vi "setTextToDocument.vi"(8 "error in (no error)":errorcluster, 11 "xwpfRun in":refnum<class "xwpfRun.lvclass">) -> (0 "error out":errorcluster, 3 "xwpfRun out":refnum<class "xwpfRun.lvclass">)   [LabVIEW 2017, in "Word_Specific.lvlib" / "xwpfRun.lvclass"]
uses:
  xwpfRun.lvclass
  xwpfRun.lvclass/xwpfRun.ctl
  C:/Program Files (x86)/National Instruments/LabVIEW 2017/vi.lib/BenjaminR/LabVIEW NPOI/lib/NPOI 2.1.1/NPOI.OOXML.dll
  Program Files (x86)/National Instruments/LabVIEW 2017/vi.lib/BenjaminR/LabVIEW NPOI/lib/NPOI 2.1.1/NPOI.OOXML.dll
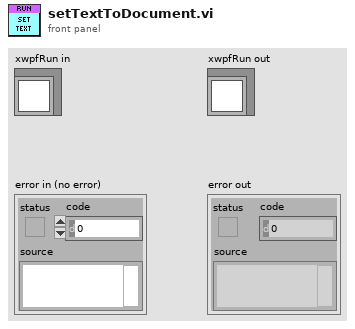
[diagram p1: front panel]
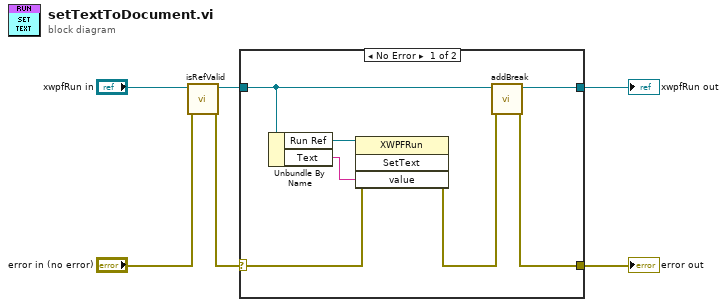
[diagram p0: block diagram]
diagram:
  n1 = call-dynamic "isRefValid.vi"("error in (no error)"="error in (no error)", "xwpfRun in"="xwpfRun in") -> ("error out"=w1:errorcluster, "xwpfRun out"=w3:refnum<class "xwpfRun.lvclass">)  [unwired: 8 in]
  n2 = case shown="No Error" w1 {
    selector: w1 -> [w11 w15]
    tunnel: [w7 w15] -> w6
    tunnel: [w9 w14] -> w4
    tunnel: w3 -> [w12 w14]
    frame No Error {
      n3 = Unbundle By Name(w12) -> ("Run Ref"=w13:refnum<k24>, "Text"=w10:string)
      n4 = invoke class="XWPFRun" method="SetText"(reference=w13, error in=w11, "value"=w10) -> (error out=w8:errorcluster)  [unwired: 1 in, 3 out]
      n5 = call-dynamic "addBreak.vi"("error in (no error)"=w8, "xwpfRun in"=w12) -> ("error out"=w7:errorcluster, "xwpfRun out"=w9:refnum<class "xwpfRun.lvclass">)  [unwired: 8 in]
    }
    frame Error {
    }
  }
  "error out" <- w6
  "xwpfRun out" <- w4
